vi "Plot Points Only.vi"() -> ()   [LabVIEW 2013]
uses:
  <vilib>/Platform/NI_3dgraph.lvlib
panel:
  in  "z vector":dbl[](array[numeric]) format="%.2f"
  in  "y vector":dbl[](array[numeric]) format="%.2f"
  in  "x vector":dbl[](array[numeric]) format="%.2f"
  in  "3D Curve - Lorenz Attractor":refnum<k7>(container)
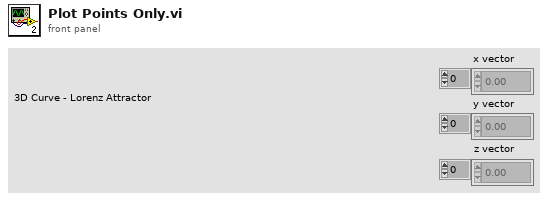
[diagram p1: front panel]
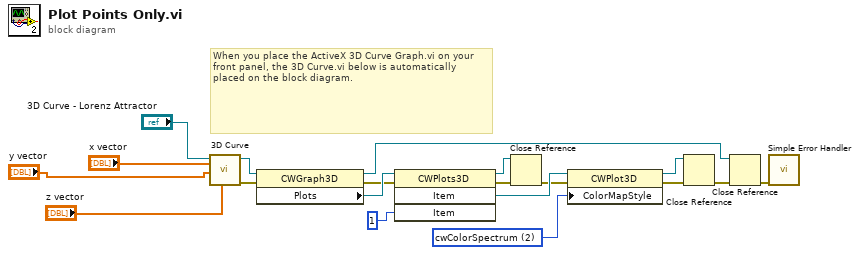
[diagram p0: block diagram]
diagram:
  w17 = 2 items=["cwNone", "cwShaded", "cwColorSpectrum", "cwGrayScale"] ("ColorMapStyle")
  # "When you place the ActiveX 3D Curve Graph.vi on your front panel, the 3D Curve.vi below is automatically placed on the block diagram."
  n1 = call <vilib>:"3D Curve.vi"("z vector"="z vector", "y vector"="y vector", "x vector"="x vector", "3D graph"="3D Curve - Lorenz Attractor") -> ("error out"=w15:errorcluster, "3D graph out"=w14:refnum<k7>)  [unwired: 6 in]
  n2 = property class="CWGraph3D"(reference=w14, error in=w15) -> (reference out=w5:refnum<k7>, error out=w13:errorcluster, "Plots"=w18:refnum<k7>)
  n3 = invoke class="CWPlots3D" method="Item"(reference=w18, error in=w13, "Item"=1) -> (reference out=w11:refnum<k7>, error out=w12:errorcluster, "Item"=w16:refnum<k7>)  [unwired: 1 in, 1 out]
  n4 = Close Reference(reference=w11, error in (no error)=w12) -> (error out=w10:errorcluster)
  n5 = property class="CWPlot3D"(reference=w16, error in=w10, "ColorMapStyle"=w17) -> (reference out=w8:refnum<k7>, error out=w9:errorcluster)
  n6 = Close Reference(reference=w8, error in (no error)=w9) -> (error out=w6:errorcluster)
  n7 = Close Reference(reference=w5, error in (no error)=w6) -> (error out=w7:errorcluster)
  n8 = call <vilib>:"Simple Error Handler.vi"("error in (no error)"=w7) -> ()  [unwired: 4 in, 5 out]
